vi "stopped.vi"(8 "error in (no error)":errorcluster, 10 "stopped":bool, 11 "PixelflySA in":refnum<class "PixelflySA.lvclass">) -> (0 "error out":errorcluster, 3 "PixelflySA out":refnum<class "PixelflySA.lvclass">)   [LabVIEW 2009, in "PixelflySA.lvclass"]
uses:
  PixelflySA.lvclass
  Channels.lvlib
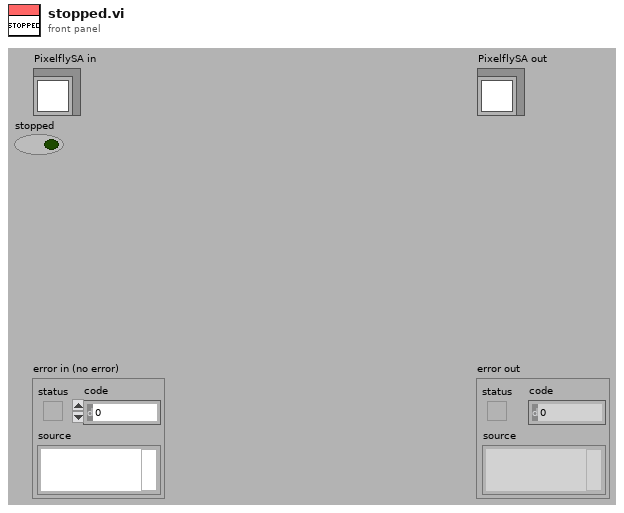
[diagram p1: front panel]
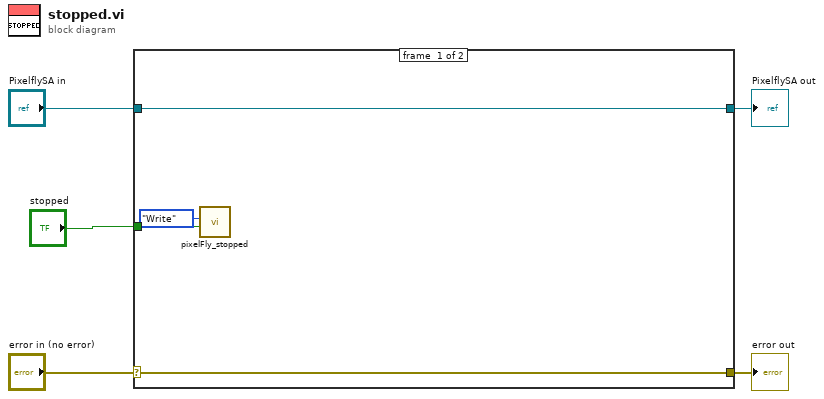
[diagram p0: block diagram]
diagram:
  n1 = case shown="No Error" "error in (no error)" {
    selector: "error in (no error)" -> [w9 w11]
    tunnel: [w9 w11] -> w4
    tunnel: [w8 w10] -> w2
    tunnel: "PixelflySA in" -> [w8 w10]
    tunnel: "stopped" -> [w7 _]
    frame #0 {
      n2 = call "pixelFly_stopped.vi"("stop"=w7, "Action"=enum16{"Write", "Read"}."Write") -> ()  [unwired: 9 in, 1 out]
    }
    frame #1 {
    }
  }
  "error out" <- w4
  "PixelflySA out" <- w2
